vi "Serialize.vi"(7 "DestinationFolder":path, 8 "error in":errorcluster, 9 "OwningElement in":refnum<k20>, 10 "Document in":refnum<k20>, 11 "ProductUnit in":refnum<class "ProductUnit.lvclass">) -> (0 "error out":errorcluster, 1 "OwningElement out":refnum<k20>, 2 "Document out":refnum<k20>, 3 "ProductUnit out":refnum<class "ProductUnit.lvclass">)   [LabVIEW 2021, in "ProligentXMLGenerator.lvlib" / "ProductUnit.lvclass"]
uses:
  ProductUnit.lvclass
  ProductUnit.lvclass/ProductUnit.ctl
  <vilib>/xml/NI_XML.lvlib
  Base/DOMSupport/DOMSupport.lvlib
  Model/CustomData/CustomData.lvclass
  Model/Document/Document.lvclass
  Model/Characteristic/Characteristic.lvclass
  <vilib>/xml/Close Reference(Node).vi
  Base/NonEmptyString_50/NonEmptyString_50.lvclass
  C:/Projects/proligent-xml-generator-labview/src/ProligentXMLGenerator/Base/NonEmptyString/NonEmptyString.lvclass
  C:/Projects/proligent-xml-generator-labview/src/ProligentXMLGenerator/Base/String/String.lvclass
  C:/Projects/proligent-xml-generator-labview/src/ProligentXMLGenerator/Base/Attribute/Attribute.lvclass
  C:/Projects/proligent-xml-generator-labview/src/ProligentXMLGenerator/Base/NonEmptyString_50/NonEmptyString_50.lvclass
  Base/FullName/FullName.lvclass
  C:/Projects/proligent-xml-generator-labview/src/ProligentXMLGenerator/Base/FullName/FullName.lvclass
  Base/Boolean/Boolean.lvclass
  C:/Projects/proligent-xml-generator-labview/src/ProligentXMLGenerator/Base/Boolean/Boolean.lvclass
  Base/DateTime/DateTime.lvclass
  C:/Projects/proligent-xml-generator-labview/src/ProligentXMLGenerator/Base/DateTime/DateTime.lvclass
  Base/NonEmptyString_255/NonEmptyString_255.lvclass
  C:/Projects/proligent-xml-generator-labview/src/ProligentXMLGenerator/Base/NonEmptyString_255/NonEmptyString_255.lvclass
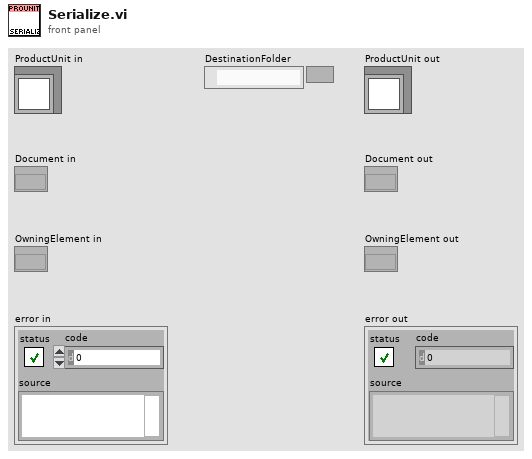
[diagram p1: front panel]
types:
  T1 = typedef "ProligentXMLGenerator.lvlib/ProductUnit.lvclass/Data.ctl" = cluster{"Name":string, "Characteristics":refnum<class "Characteristic.lvclass">[], "Documents":refnum<class "Document.lvclass">[], "CustomData":refnum<class "CustomData.lvclass">, "ProductUnitIdentifier":refnum<class "NonEmptyString_50.lvclass">, "ProductFullName":refnum<class "FullName.lvclass">, "Scrapped":refnum<class "Boolean.lvclass">, "ScrappedTime":refnum<class "DateTime.lvclass">, "CreationTime":refnum<class "DateTime.lvclass">, "ManufacturingTime":refnum<class "DateTime.lvclass">, "ByManufacturer":refnum<class "NonEmptyString_255.lvclass">, "TimeZoneInfoId":string}
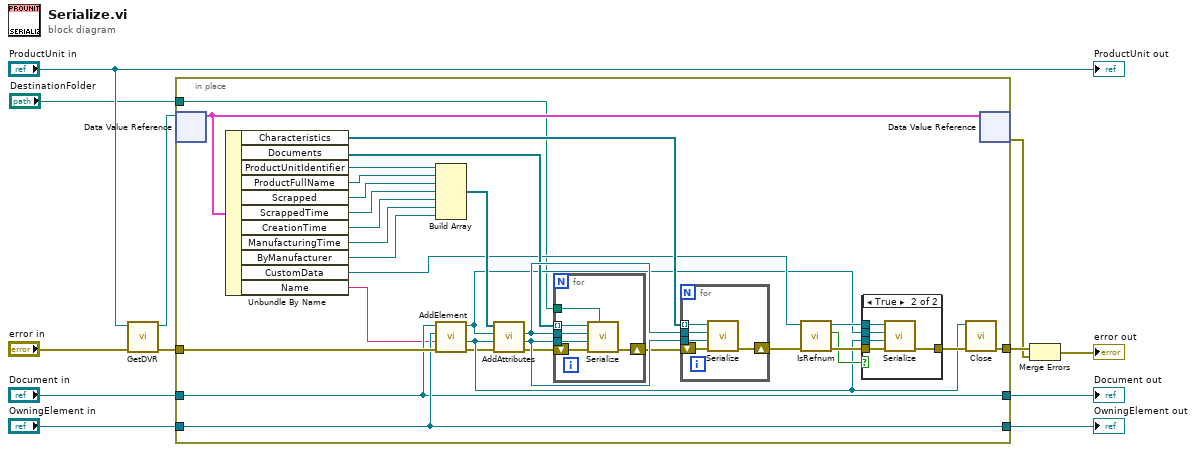
[diagram p0: block diagram]
diagram:
  n1 = call "GetDVR.vi"("error in"="error in", "ProductUnit in"="ProductUnit in") -> ("error out"=w4:errorcluster, "DVRReference"=w3:refnum<data-value>)  [unwired: 8 in]
  n2 = in-place "In Place Element Structure" {
    in-place-border: [w42] -> w5
    in-place-border: "Document in" -> [w38]
    in-place-border: w4 -> [w41]
    in-place-border: "OwningElement in" -> [w40]
    in-place-border: [w40] -> w7
    in-place-border: [w38] -> w6
    in-place-border: "DestinationFolder" -> [w13]
    n3 = in-place-dvr #1(w3) -> (w39:T1)  [unwired: 1 out]
    n4 = Unbundle By Name(w39) -> ("Characteristics"=w21:refnum<class "Characteristic.lvclass">[], "Documents"=w26:refnum<class "Document.lvclass">[], "ProductUnitIdentifier"=w31:refnum<class "NonEmptyString_50.lvclass">, "ProductFullName"=w37:refnum<class "FullName.lvclass">, "Scrapped"=w30:refnum<class "Boolean.lvclass">, "ScrappedTime"=w36:refnum<class "DateTime.lvclass">, "CreationTime"=w35:refnum<class "DateTime.lvclass">, "ManufacturingTime"=w34:refnum<class "DateTime.lvclass">, "ByManufacturer"=w33:refnum<class "NonEmptyString_255.lvclass">, "CustomData"=w18:refnum<class "CustomData.lvclass">, "Name"=w22:string)
    n5 = Build Array(w31, w37, w30, w36, w35, w34, w33) -> (w32:refnum<class "Attribute.lvclass">[])
    n6 = call "AddElement.vi"("error in"=w41, "Name"=w22, "OwningElement in"=w40, "Document in"=w38) -> ("error out"=w15:errorcluster, "NewElement"=w17:refnum<k20>, "Document out"=w16:refnum<k20>)  [unwired: 4 in, 1 out]
    n7 = call "AddAttributes.vi"("error in"=w15, "OwningElement in"=w17, "Document in"=w16, "Attributes"=w32) -> ("error out"=w14:errorcluster, "OwningElement out"=w28:refnum<k20>, "Document out"=w29:refnum<k20>)  [unwired: 5 in]
    n8 = for {
      tunnel: w26 -> [w49] mode=indexing
      tunnel: w28 -> [w52]
      tunnel: w29 -> [w53]
      shift-right: [w50] -> w27
      shift-left: w14 -> [w51]
      tunnel: w13 -> [w48]
      n9 = call "Serialize.vi"("DestinationFolder"=w48, "error in"=w51, "OwningElement in"=w52, "Document in"=w53, "DocumentType in"=w49) -> ("error out"=w50:errorcluster)  [unwired: 3 in, 3 out]
    }
    n10 = for {
      tunnel: w28 -> [w43]
      tunnel: w29 -> [w44]
      shift-right: [w46] -> w20
      shift-left: w27 -> [w47]
      tunnel: w21 -> [w45] mode=indexing
      n11 = call "Serialize.vi"("error in"=w47, "OwningElement in"=w43, "Document in"=w44, "DocumentType in"=w45) -> ("error out"=w46:errorcluster)  [unwired: 4 in, 3 out]
    }
    n12 = call "IsRefnum.vi"("error in"=w20, "CustomDataType in"=w18) -> ("error out"=w25:errorcluster, "IsRefnum"=w23:bool, "CustomDataType out"=w24:refnum<class "CustomData.lvclass">)  [unwired: 7 in]
    n13 = case shown="True" w23 {
      tunnel: w16 -> [_ w56]
      tunnel: w25 -> [w54 w59]
      tunnel: [w54 w58] -> w19
      tunnel: w24 -> [_ w57]
      tunnel: w17 -> [_ w55]
      frame False {
      }
      frame True {
        n14 = call "Serialize.vi"("error in"=w59, "OwningElement in"=w55, "Document in"=w56, "CustomDataType in"=w57) -> ("error out"=w58:errorcluster)  [unwired: 4 in, 3 out]
      }
    }
    n15 = call-poly <vilib>:"Close.vi"("error in (no error)"=w19, "node"=w17) -> ("error out"=w42:errorcluster)  [unwired: 7 in]
    n16 = in-place-dvr #1(w39) -> (w2:errorcluster)  [unwired: 1 out]
  }
  "Document out" <- w6
  "OwningElement out" <- w7
  n17 = Merge Errors(w5, w2) -> (→"error out":errorcluster)
  "ProductUnit out" <- "ProductUnit in"
